vi "SetHistoryLength.vi"(7 "LabVIEW Web Service Request":refnum<class "Web Request.lvclass">) -> ()   [LabVIEW 2018]
uses:
  <vilib>/wsapi/Web Request.lvclass
  CAEN globals.vi
panel:
  in  "error in (no error)":errorcluster
  # "Use the Web Service Request input terminal to call the VIs on the Web Services palette. Do not remove it from the connector pane unless you don't need access to the palette."
  # "Each additional control wired to the connector pane will be available as an input in the URL. To include an indicator in terminal-mode output (the default setting), it must also be wired to the connector pane."
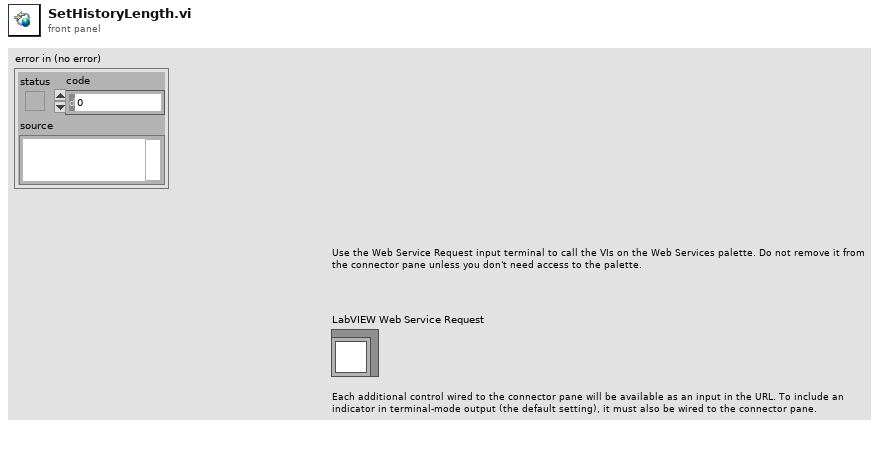
[diagram p1: front panel]
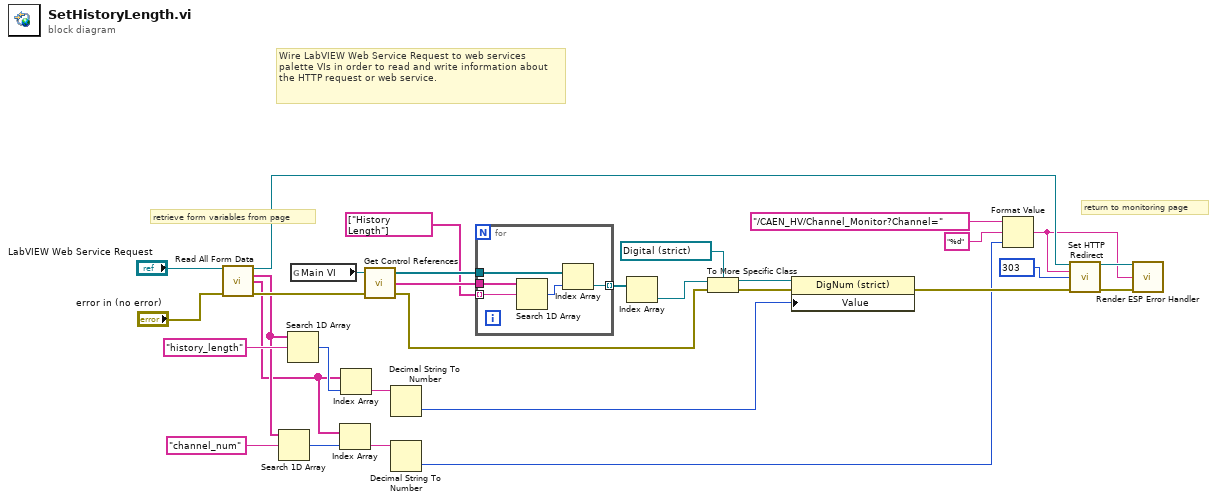
[diagram p0: block diagram]
diagram:
  w28 = 303 items=["100"=100, "101"=101, "200"=200, "201"=201, "202"=202, "203"=203, "204"=204, "205"=205, "206"=206, "300"=300, "301"=301, "302"=302, "303"=303, "304"=304, "305"=305, "306"=306, "307"=307, "400"=400, "401"=401, "402"=402, "403"=403, "404"=404, "405"=405, "406"=406, "407"=407, "408"=408, "409"=409, "410"=410, "411"=411, "412"=412, "413"=413, "414"=414, "415"=415, "416"=416, "417"=417, "500"=500, "501"=501, "502"=502, "503"=503, "504"=504, "505"=505] ("response code (307)")
  # "retrieve form variables from page"
  # "return to monitoring page"
  # "Wire LabVIEW Web Service Request to web services palette VIs in order to read and write information about the HTTP request or web service."
  n1 = call <vilib>:"Read All Form Data.vi"("LabVIEW Web Service Request"="LabVIEW Web Service Request", "error in (no error)"="error in (no error)") -> ("LabVIEW Web Service Request out"=w23:refnum<class "Web Request.lvclass">, "Key"=w11:string[], "Value"=w9:string[], "error out"=w24:errorcluster)  [unwired: 9 in, 1 out]
  n2 = Search 1D Array(1D array=w11, element="channel_num") -> (index of element=w8:i32)  [unwired: 1 in]
  n3 = Search 1D Array(1D array=w11, element="history_length") -> (index of element=w18:i32)  [unwired: 1 in]
  n4 = global read "CAEN globals.vi" "Main VI"() -> (w31:refnum<vi>)
  n5 = Index Array(array=w9, index=w8) -> (element=w6:string)
  n6 = Index Array(array=w9, index=w18) -> (element=w17:string)
  n7 = call "Get Control References.vi"("error in"=w24, "This vi"=w31) -> ("error out"=w16:errorcluster, "Control Names"=w30:string[], "Controls[]"=w29:refnum<vi>[])  [unwired: 1 in]
  n8 = Decimal String To Number(string=w17) -> (number=w7:i32)  [unwired: 2 in, 1 out]
  n9 = Decimal String To Number(string=w6) -> (number=w3:i32)  [unwired: 2 in, 1 out]
  n10 = for {
    tunnel: w30 -> [w36]
    tunnel: w29 -> [w35]
    tunnel: [w33] -> w20 mode=indexing
    tunnel: string[] ["History Length"] ("Value") -> [w32] mode=indexing
    n11 = Search 1D Array(1D array=w36, element=w32) -> (index of element=w34:i32)  [unwired: 1 in]
    n12 = Index Array(array=w35, index=w34) -> (element=w33:refnum<vi>)
  }
  n13 = Index Array(array=w20) -> (element=w19:refnum<vi>)  [unwired: 1 in]
  n14 = To More Specific Class(target class=refnum<vi> refnum ("History Length"), reference=w19, error in=w16) -> (specific class reference=w13:refnum<vi>, error out=w14:errorcluster)
  n15 = property class="DigNum (strict)"(reference=w13, error in=w14, "Value"=w7) -> (error out=w12:errorcluster)  [unwired: 1 out]
  n16 = Format Value(string ("")="/CAEN_HV/Channel_Monitor?Channel=" ("redirect URL"), format string="%d", value (0)=w3) -> (output string=w2:string)
  n17 = call <vilib>:"Set HTTP Redirect.vi"("LabVIEW Web Service Request"=w23, "redirect URL"=w2, "response code (307)"=w28, "error in (no error)"=w12) -> ("LabVIEW Web Service Request out"=w26:refnum<class "Web Request.lvclass">, "error out"=w27:errorcluster)  [unwired: 10 in]
  n18 = call "Render ESP Error Handler.vi"("LabVIEW Web Service Request"=w26, "Link"=w2, "error in (no error)"=w27) -> ()  [unwired: 11 in, 2 out]
